vi "Main.vi"() -> ()   [LabVIEW 2013]
doc: "This template is for the Queued Message Handler design pattern.\n\nThe Event Handling Loop generates messages based on user interface actions.\n\nThe Message Handling Loop processes messages generated by the Event Handling Loop, or by other messages. The messages are string values, so new messages can be added easily to the Message Cases case structure in the Message Handling Loop. Each message cluster can also provide an optional value for Message Data, which is a variant that can be converted to whatever message-specific data is required."
uses:
  controls/UI Data.ctl
  <vilib>/vision/Image Controls.llb/IMAQ Image.ctl
  support/Message Queue/Message Queue.lvlib
  support/User Event - Stop/User Event - Stop.lvlib
  support/FPGA/FPGA Frame Grabbing.lvlib
  <vilib>/vision/NI_Vision_Development_Module.lvlib
  support/Image Processing/Image Processing.lvlib
panel:
  out "combo mask":T1(plugin-control)
  out "right \nannulus":T2 {"End Angle" format="%.2f"; "Start Angle" format="%.2f"; "Center X" scale=0.0..1024.0}
  out "right masked image":T1(plugin-control)
  out "right mask":T1(plugin-control)
  out "left annulus":T2 {"End Angle" format="%.2f"; "Start Angle" format="%.2f"; "Center X" scale=0.0..1024.0}
  out "left masked image":T1(plugin-control)
  out "left mask":T1(plugin-control)
  in  "Accept Threshold":bool
  in  "Threshold Range":cluster{"Lower value":dbl, "Upper value":dbl}={"Lower value"=0.0, "Upper value"=255.0} {"Upper value" min=0.0 max=255.0 scale=0.0..255.0; "Lower value" min=0.0 max=255.0 scale=0.0..255.0}
  out "FPGA image info":T5 {"Image Type" items=["Grayscale (U8)", "Grayscale (I16)", "Grayscale (SGL)", "Complex (CSG)", "RGB (U32)", "HSL (U32)", "RGB (U64)", "Grayscale (U16)"]}
  out "Processed Image":T1(plugin-control)
  in  "Stream?":bool
  out "FPGA Image":T1(plugin-control)
  in  "Save Mask Coordinates":bool
  in  "Test Visual Response":bool
  in  "Send Parameters to FPGA":bool
  out "Status Update":string="VI Stopped"
  in  "Define Mask":bool
  in  "Acquire Image":bool
  in  "Stop":bool
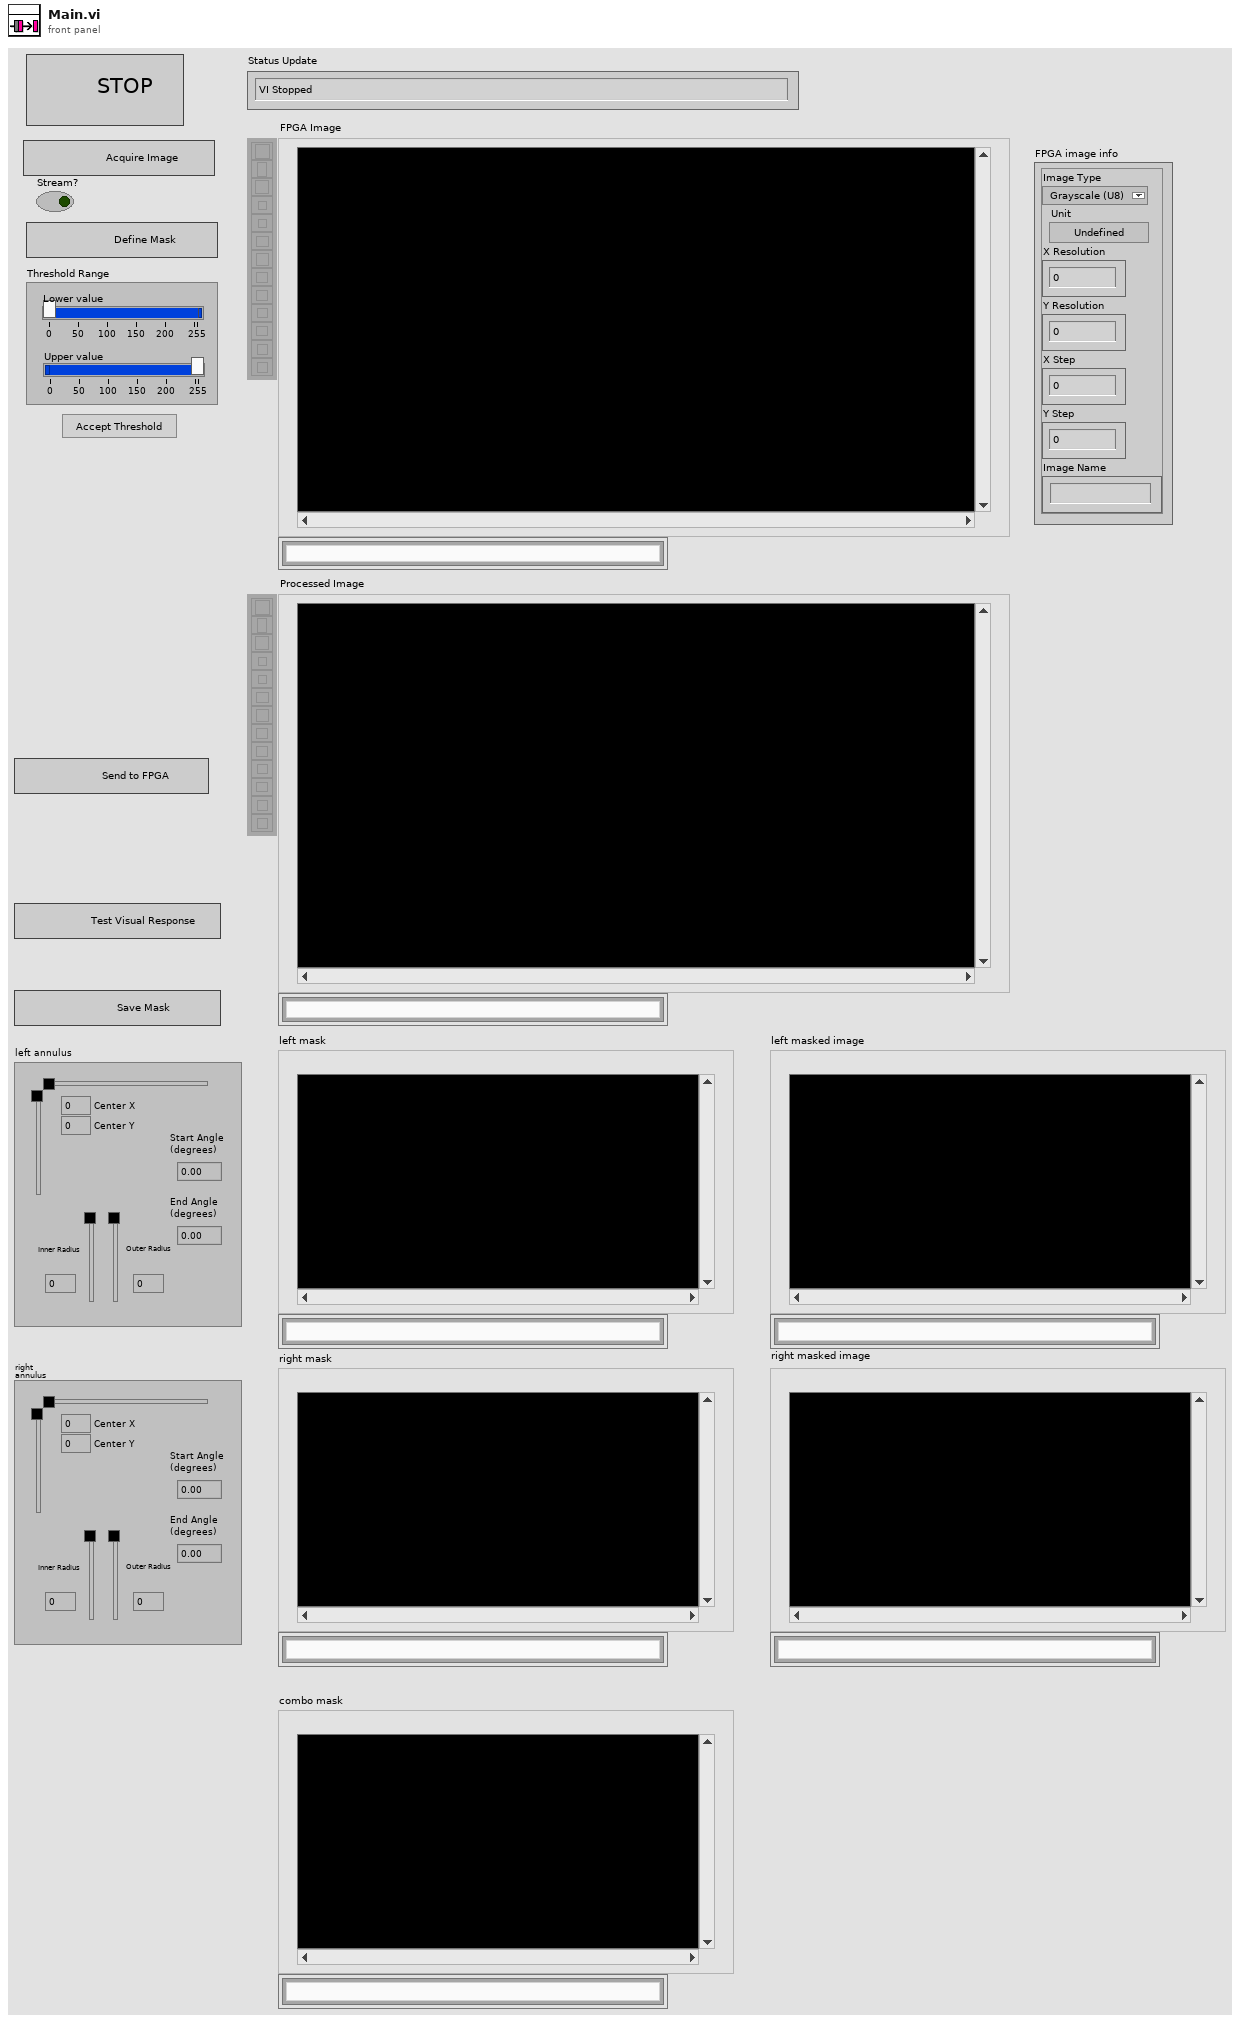
[diagram p1: front panel]
types:
  T1 = typedef "IMAQ Image.ctl" = refnum<image>
  T2 = typedef "IMAQ Circle" = cluster{"Center X":i32, "Center Y":i32, "Inner Radius":i32, "Outer Radius":i32, "Start Angle":dbl, "End Angle":dbl}
  T3 = typedef "Image Type" = u32
  T4 = typedef "Image Unit" = enum32{"Undefined", "Angström", "Micrometer", "Millimeter", "Centimeter", "Meter", "Kilometer", "Microinch", "Inch", "Feet", "Nautical miles", "Standard miles", "Steps"}
  T5 = cluster{"Image Type":T3, "Unit":T4, "X Resolution":i32, "Y Resolution":i32, "X Step":sgl, "Y Step":sgl, "Image Name":string}
  T6 = typedef "UI Data.ctl" = cluster{"Boolean <Replace Me>":bool, "Initial Message":string, "Numeric <Replace Me>":dbl, "Acquire Image Ref":refnum<vi>, "Define Mask Ref":refnum<vi>, "Status Update Ref":refnum<vi>, "Stop Button Ref":refnum<vi>, "FPGA Image":T1, "Processed Image":T1, "Left Annulus":cluster{"Center X":i32, "Center Y":i32, "Inner Radius":i32, "Outer Radius":i32, "Start Angle":dbl, "End Angle":dbl}, "Right Annulus":cluster{"Center X":i32, "Center Y":i32, "Inner Radius":i32, "Outer Radius":i32, "Start Angle":dbl, "End Angle":dbl}}
  T7 = typedef "Message Queue.lvlib/All Message Queues.ctl" = cluster{"UI":refnum<queue>}
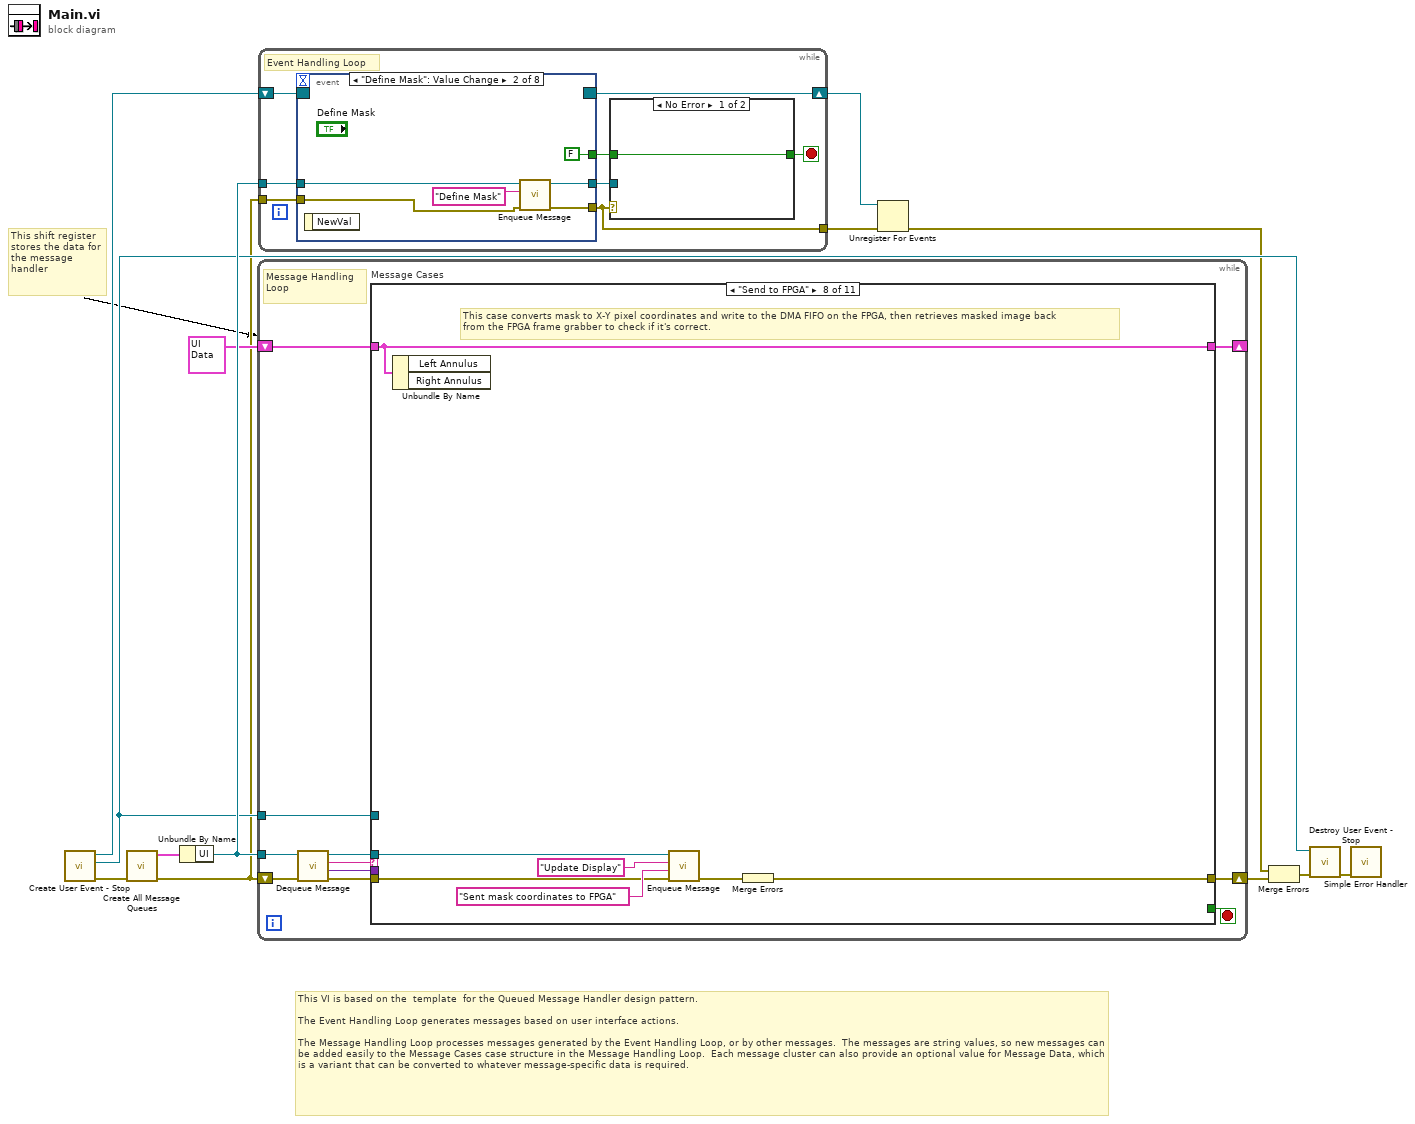
[diagram p0: block diagram]
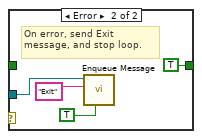
[diagram p2: hidden frame]
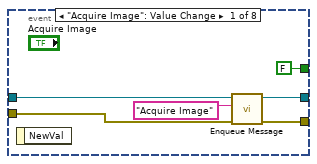
[diagram p3: hidden frame]
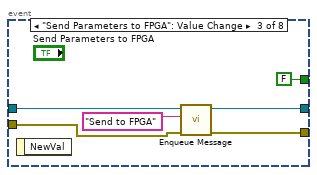
[diagram p4: hidden frame]
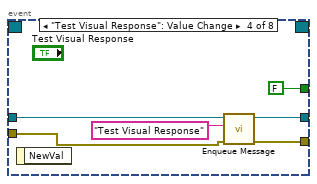
[diagram p5: hidden frame]
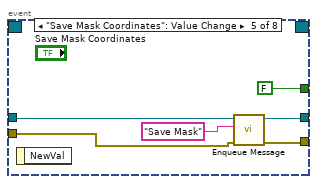
[diagram p6: hidden frame]
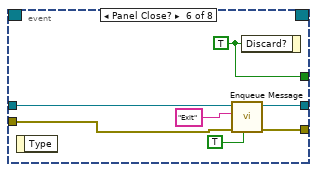
[diagram p7: hidden frame]
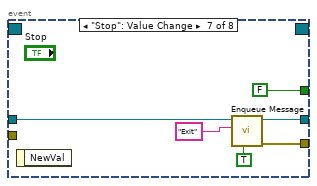
[diagram p8: hidden frame]
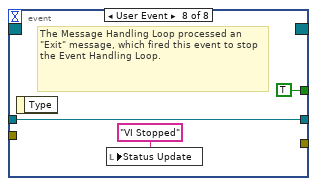
[diagram p9: hidden frame]
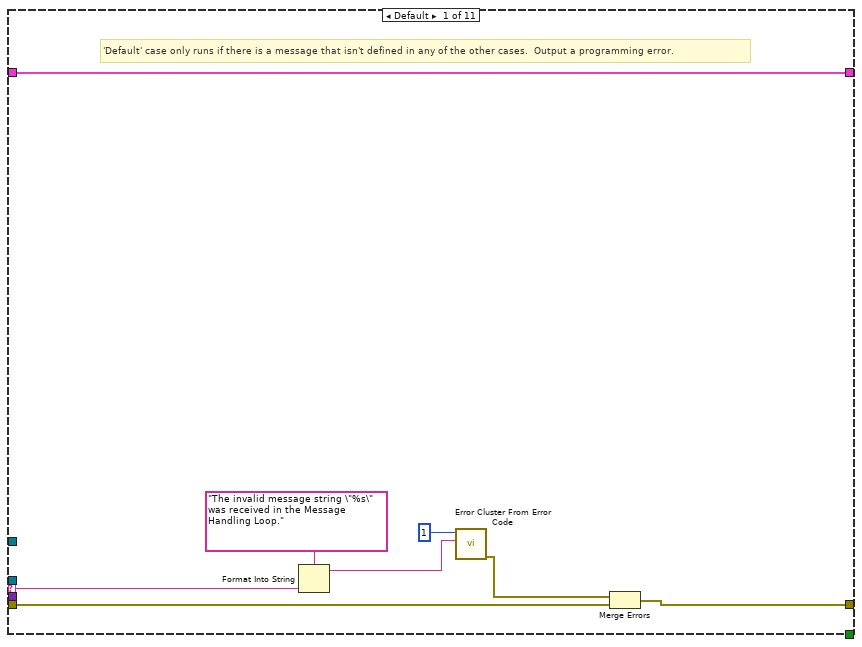
[diagram p10: hidden frame]
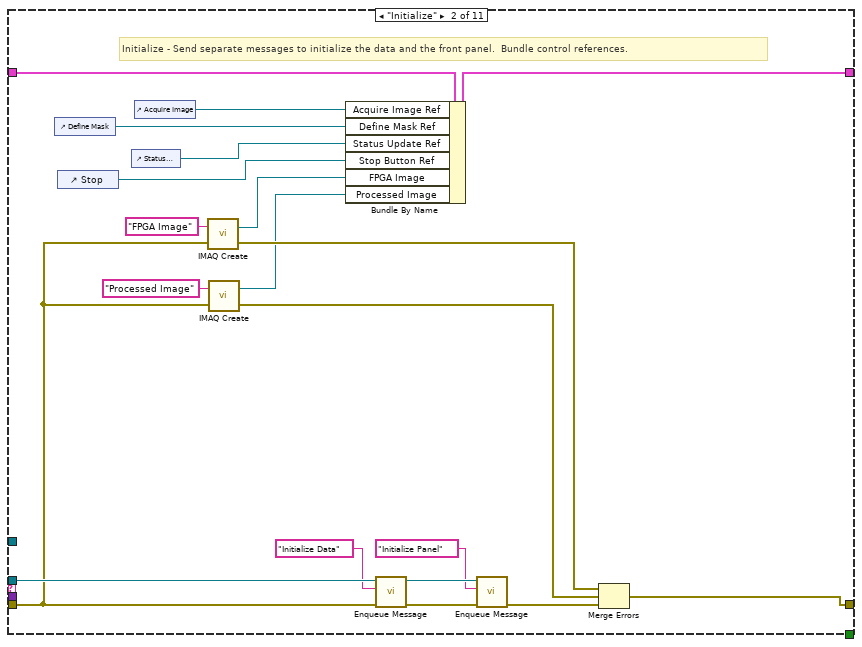
[diagram p11: hidden frame]
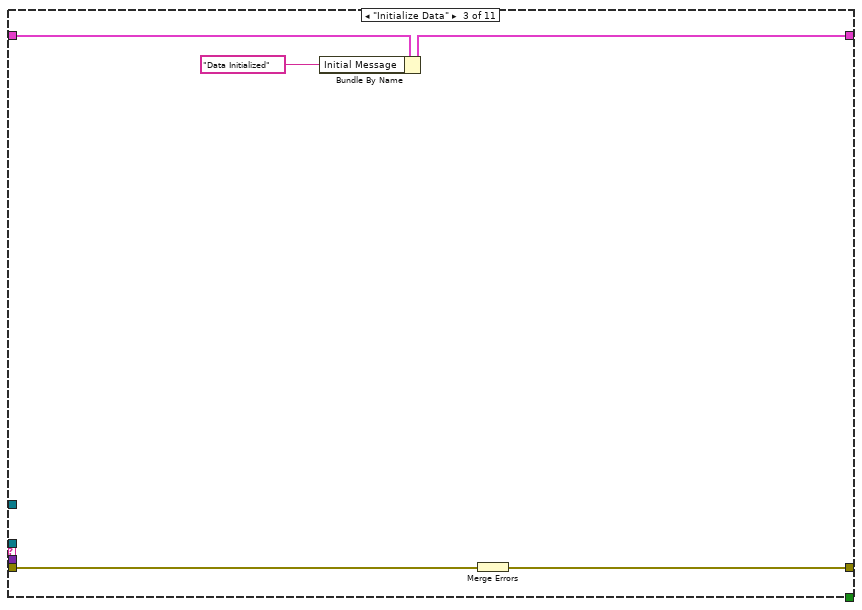
[diagram p12: hidden frame]
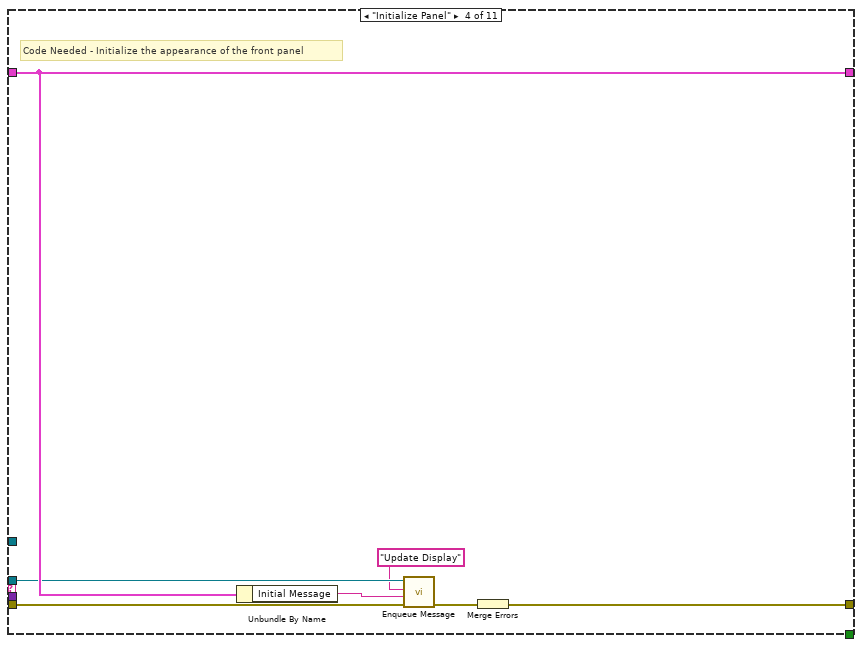
[diagram p13: hidden frame]
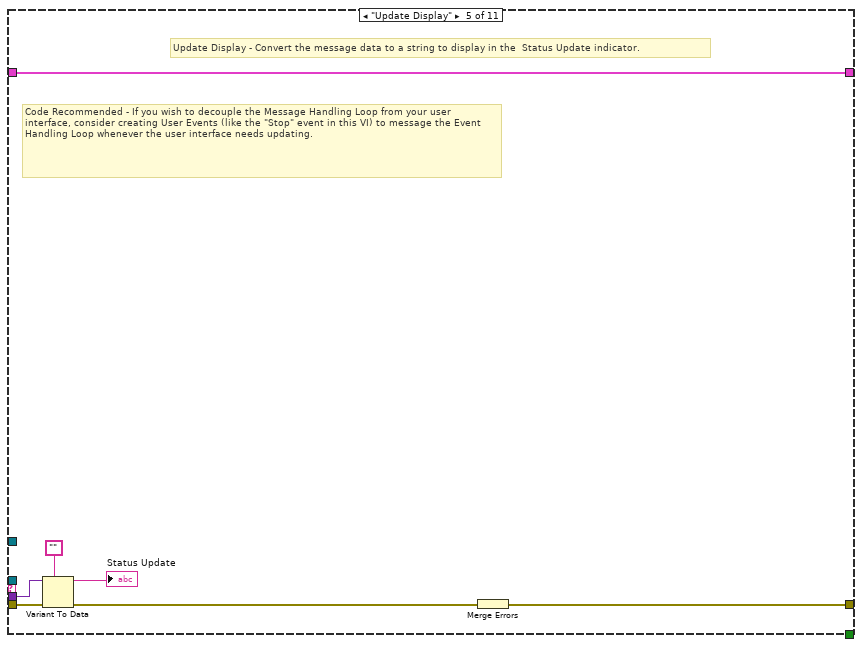
[diagram p14: hidden frame]
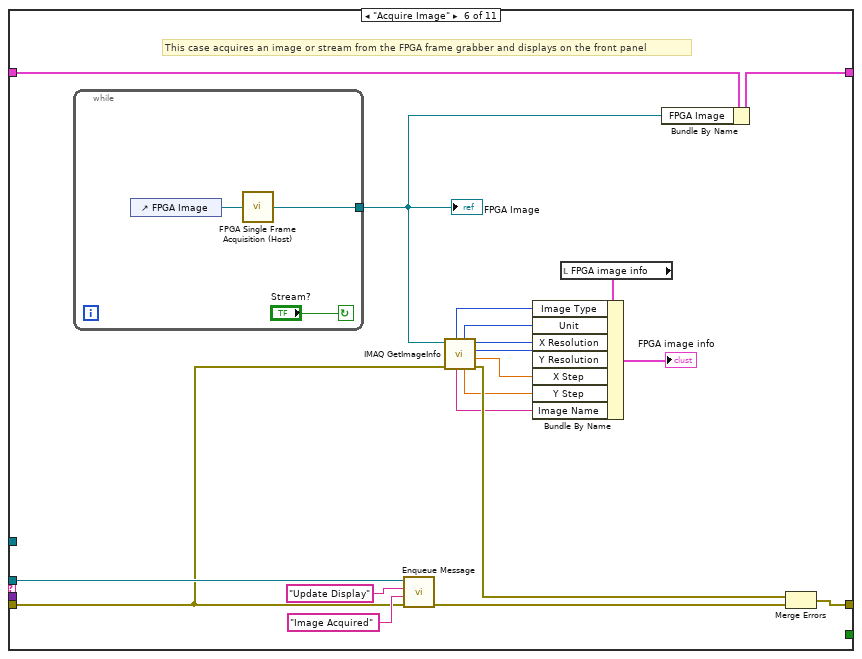
[diagram p15: hidden frame]
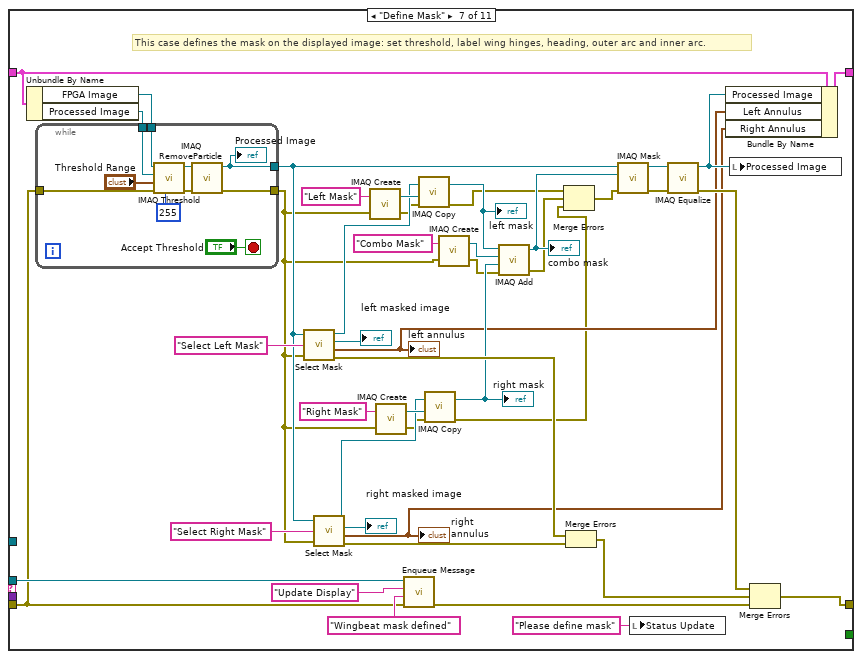
[diagram p16: hidden frame]
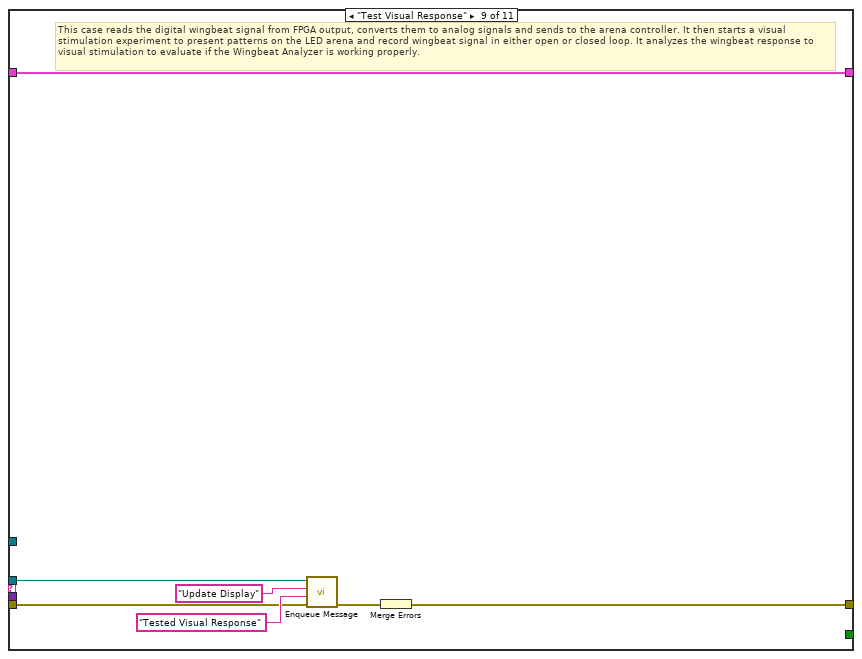
[diagram p17: hidden frame]
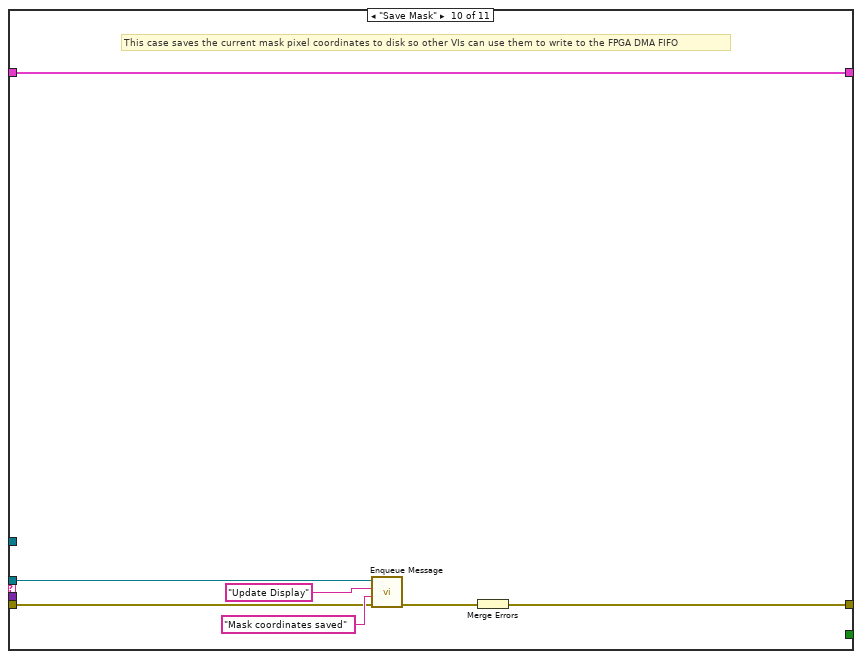
[diagram p18: hidden frame]
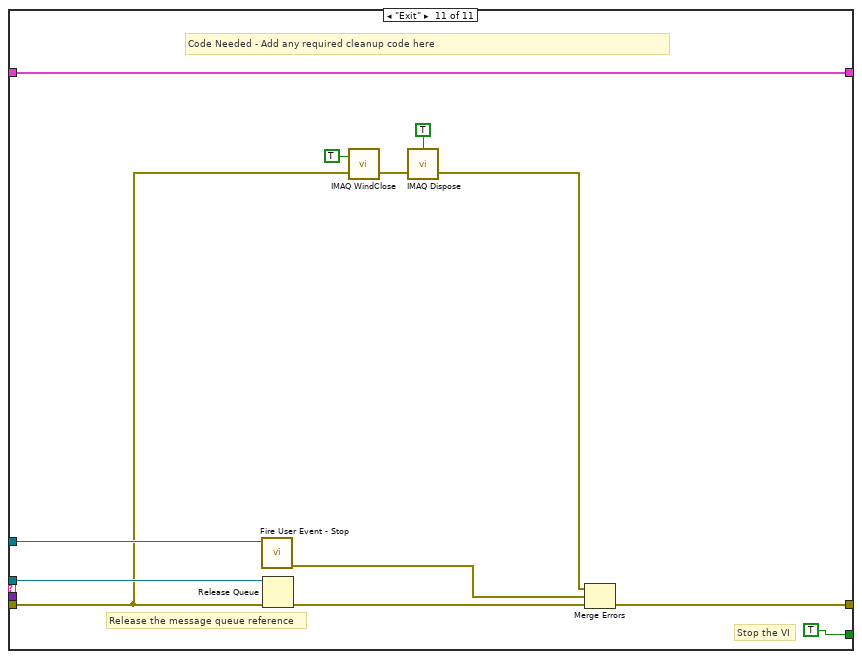
[diagram p19: hidden frame]
diagram:
  # "This VI is based on the  template  for the Queued Message Handler design pattern.\n\nThe Event Handling Loop generates messages based on user interface actions.\n\nThe Message Handling Loop processes messages generated by the Event Handling Loop, or by other messages.  The messages are string values, so new messages can be added easily to the Message Cases case structure in the Message Handling Loop.  Each message cluster can also provide an optional value for Message Data, which is a variant that can be converted to whatever message-specific data is required."
  # "This shift register\nstores the data for the message handler"
  n1 = call "Create User Event - Stop.vi"() -> ("error out"=w9:errorcluster, "User Event - Stop"=w6:refnum<user-event>, "Stop Event Registration Refnum"=w10:refnum<event-registration>)  [unwired: 9 in]
  n2 = call "Create All Message Queues.vi"("error in (no error)"=w9) -> ("error out"=w1:errorcluster, "Message Queues out"=w13:T7)  [unwired: 9 in]
  n3 = Unbundle By Name(w13) -> ("UI"=w11:refnum<queue>)
  n4 = while {
    tunnel: w11 -> [w14]
    shift-right: [w23] -> _
    shift-left: T6 {"Boolean <Replace Me>"=TRUE, "Initial Message"="", "Numeric <Replace Me>"=0.0, "Acquire Image Ref"=refnum, "Define Mask Ref"=refnum, "Status Update Ref"=refnum, "Stop Button Ref"=refnum, "FPGA Image"=refnum, "Processed Image"=refnum, "Left Annulus"={"Center X"=0, "Center Y"=0, "Inner Radius"=0, "Outer Radius"=0, "Start Angle"=0.0, "End Angle"=0.0}, "Right Annulus"={"Center X"=0, "Center Y"=0, "Inner Radius"=0, "Outer Radius"=0, "Start Angle"=0.0, "End Angle"=0.0}} ("Data Cluster") -> [w24]
    tunnel: w6 -> [w20]
    shift-right: [w21] -> w12
    shift-left: w1 -> [w19]
    stop <- w22 stop-if-true
    # "Message Handling Loop"
    n5 = call "Dequeue Message.vi"("error in (no error)"=w19, "Message Queue"=w14) -> ("error out"=w18:errorcluster, "Message Data"=w16:variant, "Message"=w17:string, "dup Message Queue"=w15:refnum<queue>)  [unwired: 6 in]
    n6 = case "Message Cases" shown="\"Send to FPGA\"" w17 {
      selector: w17 -> [w30 _ _ _ _ _ _ _ _ _ _]
      tunnel: w15 -> [_ w50 _ w61 _ w88 w137 w150 w156 w164 w180]
      tunnel: w18 -> [w27 w35 w57 w62 w69 w83 w134 w151 w157 w162 w169]
      tunnel: [w25 w37 w53 w63 w70 w90 w94 w149 w155 w167 w176] -> w21
      tunnel: w24 -> [w32 w47 w56 w64 w71 w85 w133 w148 w161 w168 w179]
      tunnel: [w32 w46 w55 w64 w71 w84 w132 w148 w161 w168 w179] -> w23
      tunnel: [_ _ _ _ _ _ _ _ _ _ TRUE] -> w22
      tunnel: w16 -> [_ _ _ _ w68 _ _ _ _ _ _]
      tunnel: w20 -> [_ _ _ _ _ _ _ _ _ _ w175]
      frame Default {
        # "'Default' case only runs if there is a message that isn't defined in any of the other cases.  Output a programming error."
        n7 = Format Into String(format string="The invalid message string \"%s\" was received in the Message Handling Loop." ("Unknown Message Error Text"), w30) -> (resulting string=w28:string)  [unwired: 2 in, 1 out]
        n8 = call <vilib>:"Error Cluster From Error Code.vi"("error message (\"\")"=w28, "error code (0)"=1) -> ("error out"=w26:errorcluster)  [unwired: 7 in]
        n9 = Merge Errors(w26, w27) -> (w25:errorcluster)
      }
      frame "Initialize" {
        # "Initialize - Send separate messages to initialize the data and the front panel.  Bundle control references."
        n10 = control-ref of="Define Mask"() -> (w44:refnum<vi>)
        n11 = control-ref of="Stop"() -> (w42:refnum<vi>)
        n12 = control-ref of="Status Update"() -> (w43:refnum<vi>)
        n13 = control-ref of="Acquire Image"() -> (w45:refnum<vi>)
        n14 = call "IMAQ Create"("Image Name"="FPGA Image", "error in (no error)"=w35) -> ("New Image"=w40:T1, "error out"=w36:errorcluster)  [unwired: 3 in]
        n15 = call "IMAQ Create"("Image Name"="Processed Image", "error in (no error)"=w35) -> ("New Image"=w33:T1, "error out"=w34:errorcluster)  [unwired: 3 in]
        n16 = Bundle By Name(cluster=w47, "Acquire Image Ref"=w45, "Define Mask Ref"=w44, "Status Update Ref"=w43, "Stop Button Ref"=w42, "FPGA Image"=w40, "Processed Image"=w33) -> (w46:T6)
        n17 = call "Enqueue Message.vi"("error in (no error)"=w35, "Message"="Initialize Data", "Message Queue"=w50) -> ("error out"=w52:errorcluster, "dup Message Queue"=w51:refnum<queue>)  [unwired: 7 in]
        n18 = call "Enqueue Message.vi"("error in (no error)"=w52, "Message"="Initialize Panel", "Message Queue"=w51) -> ("error out"=w38:errorcluster)  [unwired: 7 in, 1 out]
        n19 = Merge Errors(w36, w34, w38) -> (w37:errorcluster)
      }
      frame "Initialize Data" {
        n20 = Bundle By Name(cluster=w56, "Initial Message"="Data Initialized") -> (w55:T6)
        n21 = Merge Errors(w57) -> (w53:errorcluster)
      }
      frame "Initialize Panel" {
        # "Code Needed - Initialize the appearance of the front panel"
        n22 = Unbundle By Name(w64) -> ("Initial Message"=w58:string)
        n23 = call "Enqueue Message.vi"("error in (no error)"=w62, "Message Data"=w58, "Message"="Update Display", "Message Queue"=w61) -> ("error out"=w60:errorcluster)  [unwired: 6 in, 1 out]
        n24 = Merge Errors(w60) -> (w63:errorcluster)
      }
      frame "Update Display" {
        # "Code Recommended - If you wish to decouple the Message Handling Loop from your user interface, consider creating User Events (like the \"Stop\" event in this VI) to message the Event Handling Loop whenever the user interface needs updating."
        # "Update Display - Convert the message data to a string to display in the  Status Update indicator."
        n25 = Variant To Data(error in=w69, type="", Variant=w68) -> (data=→"Status Update":string, error out=w66:errorcluster)
        n26 = Merge Errors(w66) -> (w70:errorcluster)
      }
      frame "Acquire Image" {
        # "This case acquires an image or stream from the FPGA frame grabber and displays on the front panel"
        n27 = while {
          tunnel: [w92] -> w72
          stop <- "Stream?" continue-if-true
          n28 = control-ref of="FPGA Image"() -> (w91:refnum<vi>)
          n29 = call "FPGA Single Frame Acquisition (Host).vi"("Ctl Refnum"=w91) -> ("Image"=w92:T1)
        }
        "FPGA Image" <- w72
        n30 = call "Enqueue Message.vi"("error in (no error)"=w83, "Message Data"="Image Acquired" ("\"Do Something\" button pressed"), "Message"="Update Display", "Message Queue"=w88) -> ("error out"=w89:errorcluster)  [unwired: 6 in, 1 out]
        n31 = call "IMAQ GetImageInfo"("error in (no error)"=w83, "Image"=w72) -> ("error out"=w82:errorcluster, "X Step"=w77:sgl, "Y Resolution"=w78:i32, "X Resolution"=w79:i32, "Y Step"=w76:sgl, "Unit"=w80:T4, "Image Name"=w75:string, "Image Type"=w81:T3)  [unwired: 2 in]
        n32 = local read "FPGA image info"() -> (w73:T5)
        n33 = Bundle By Name(cluster=w73, "Image Type"=w81, "Unit"=w80, "X Resolution"=w79, "Y Resolution"=w78, "X Step"=w77, "Y Step"=w76, "Image Name"=w75) -> (→"FPGA image info":T5)
        n34 = Bundle By Name(cluster=w85, "FPGA Image"=w72) -> (w84:T6)
        n35 = Merge Errors(w82, w89) -> (w90:errorcluster)
      }
      frame "Define Mask" {
        # "This case defines the mask on the displayed image: set threshold, label wing hinges, heading, outer arc and inner arc."
        n36 = Unbundle By Name(w133) -> ("FPGA Image"=w131:T1, "Processed Image"=w130:T1)
        n37 = while {
          tunnel: w134 -> [w147]
          tunnel: w131 -> [w146]
          tunnel: w130 -> [w145]
          tunnel: [w138] -> w116
          tunnel: [w140] -> w100
          stop <- "Accept Threshold" stop-if-true
          n38 = call "IMAQ Threshold"("Replace Value"=u8 255, "error in (no error)"=w147, "Range"="Threshold Range", "Image Dst"=w145, "Image Src"=w146) -> ("error out"=w143:errorcluster, "Image Dst Out"=w142:T1)  [unwired: 1 in, 4 out]
          n39 = call "IMAQ RemoveParticle"("error in (no error)"=w143, "Image Src"=w142) -> ("error out"=w140:errorcluster, "Image Dst Out"=w138:T1)  [unwired: 5 in, 3 out]
          "Processed Image" <- w138
        }
        n40 = call "Select Mask.vi"("Read \nImage"=w116, "Prompt"="Select Left Mask", "error in"=w100) -> ("mask"=w109:T1, "Masked \nImage"=→"left masked image":T1, "Annulus"=w105:T2, "error out"=w120:errorcluster)  [unwired: 1 out]
        "left annulus" <- w105
        n41 = call "Select Mask.vi"("Read \nImage"=w116, "Prompt"="Select Right Mask", "error in"=w100) -> ("mask"=w107:T1, "Masked \nImage"=→"right masked image":T1, "Annulus"=w104:T2, "error out"=w119:errorcluster)  [unwired: 1 out]
        "right \nannulus" <- w104
        n42 = call "IMAQ Create"("Image Name"="Left Mask", "error in (no error)"=w100) -> ("New Image"=w112:T1, "error out"=w103:errorcluster)  [unwired: 3 in]
        n43 = call "IMAQ Create"("Image Name"="Right Mask", "error in (no error)"=w100) -> ("New Image"=w110:T1, "error out"=w102:errorcluster)  [unwired: 3 in]
        n44 = call "Enqueue Message.vi"("error in (no error)"=w134, "Message Data"="Wingbeat mask defined" ("\"Do Something Else\" button pressed"), "Message"="Update Display", "Message Queue"=w137) -> ("error out"=w95:errorcluster)  [unwired: 6 in, 1 out]
        n45 = call "IMAQ Copy"("error in (no error)"=w103, "Image Dst"=w112, "Image Src"=w109) -> ("error out"=w99:errorcluster, "Image Dst Out"=w108:T1)  [unwired: 3 in]
        "left mask" <- w108
        n46 = call "IMAQ Copy"("error in (no error)"=w102, "Image Dst"=w110, "Image Src"=w107) -> ("error out"=w97:errorcluster, "Image Dst Out"=w106:T1)  [unwired: 3 in]
        "right mask" <- w106
        n47 = call "IMAQ Create"("Image Name"="Combo Mask", "error in (no error)"=w100) -> ("New Image"=w117:T1, "error out"=w101:errorcluster)  [unwired: 3 in]
        n48 = call "IMAQ Add"("Image Src A"=w108, "Image Dst"=w117, "Image Src B"=w106, "error in (no error)"=w101) -> ("Image Dst Out"=w114:T1, "error out"=w98:errorcluster)  [unwired: 3 in]
        "combo mask" <- w114
        n49 = Merge Errors(w99, w98, w97) -> (w96:errorcluster)
        n50 = Merge Errors(w120, w119) -> (w115:errorcluster)
        n51 = call "IMAQ Mask"("error in (no error)"=w96, "Image Mask"=w114, "Image Src"=w116) -> ("error out"=w125:errorcluster, "Image Dst Out"=w126:T1)  [unwired: 1 in, 1 out]
        n52 = local write "Status Update"("Please define mask" ("Status Update")) -> ()
        n53 = call "IMAQ Equalize"("error in (no error)"=w125, "Image Src"=w126) -> ("error out"=w128:errorcluster, "Image Dst Out"=w124:T1)  [unwired: 4 in, 4 out]
        n54 = Bundle By Name(cluster=w133, "Processed Image"=w124, "Left Annulus"=w105, "Right Annulus"=w104) -> (w132:T6)
        n55 = local write "Processed Image"(w124) -> ()
        n56 = Merge Errors(w128, w115, w95) -> (w94:errorcluster)
      }
      frame "Send to FPGA" {
        # "This case converts mask to X-Y pixel coordinates and write to the DMA FIFO on the FPGA, then retrieves masked image back \nfrom the FPGA frame grabber to check if it's correct."
        n57 = Unbundle By Name(w148) -> ()  [unwired: 2 out]
        n58 = call "Enqueue Message.vi"("error in (no error)"=w151, "Message Data"="Sent mask coordinates to FPGA" ("\"Do Something\" button pressed"), "Message"="Update Display", "Message Queue"=w150) -> ("error out"=w154:errorcluster)  [unwired: 6 in, 1 out]
        n59 = Merge Errors(w154) -> (w149:errorcluster)
      }
      frame "Test Visual Response" {
        # "This case reads the digital wingbeat signal from FPGA output, converts them to analog signals and sends to the arena controller. It then starts a visual stimulation experiment to present patterns on the LED arena and record wingbeat signal in either open or closed loop. It analyzes the wingbeat response to visual stimulation to evaluate if the Wingbeat Analyzer is working properly."
        n60 = call "Enqueue Message.vi"("error in (no error)"=w157, "Message Data"="Tested Visual Response" ("\"Do Something\" button pressed"), "Message"="Update Display", "Message Queue"=w156) -> ("error out"=w160:errorcluster)  [unwired: 6 in, 1 out]
        n61 = Merge Errors(w160) -> (w155:errorcluster)
      }
      frame "Save Mask" {
        # "This case saves the current mask pixel coordinates to disk so other VIs can use them to write to the FPGA DMA FIFO"
        n62 = call "Enqueue Message.vi"("error in (no error)"=w162, "Message Data"="Mask coordinates saved" ("\"Do Something Else\" button pressed"), "Message"="Update Display", "Message Queue"=w164) -> ("error out"=w163:errorcluster)  [unwired: 6 in, 1 out]
        n63 = Merge Errors(w163) -> (w167:errorcluster)
      }
      frame "Exit" {
        # "Stop the VI"
        # "Release the message queue reference"
        # "Code Needed - Add any required cleanup code here"
        n64 = call "Fire User Event - Stop.vi"("User Event - Stop"=w175) -> ("error out"=w174:errorcluster)  [unwired: 10 in]
        n65 = Release Queue(queue=w180, error in (no error)=w169) -> (error out=w177:errorcluster)  [unwired: 1 in, 2 out]
        n66 = call "IMAQ WindClose"("Close All Windows (False)"=TRUE, "error in (no error)"=w169) -> ("error out"=w171:errorcluster)  [unwired: 4 in]
        n67 = call "IMAQ Dispose"("All Images? (No)"=TRUE, "error in (no error)"=w171) -> ("error out"=w170:errorcluster)  [unwired: 4 in]
        n68 = Merge Errors(w170, w174, w177) -> (w176:errorcluster)
      }
    }
  }
  n69 = while {
    tunnel: w11 -> [w188]
    tunnel: [w184] -> w4
    shift-right: [w182] -> w3
    shift-left: w10 -> [w183]
    tunnel: w1 -> [w181]
    stop <- w186 stop-if-true
    # "Event Handling Loop"
    n70 = event shown="[1] \"Define Mask\": Value Change" {
      selector: w183 -> [_ _ _ _ _ _ _ _]
      dyn-events: [_ _ _ _ _ _ _ _] -> w182
      timeout: _ -> [_ _ _ _ _ _ _ _]
      tunnel: [FALSE ("Discard?") FALSE ("Discard?") FALSE ("Discard?") FALSE ("Discard?") FALSE ("Discard?") w230 FALSE ("Discard?") TRUE ("Discard?")] -> w187
      tunnel: w188 -> [w199 w205 w211 w216 w221 w229 w236 w239]
      tunnel: [w198 w203 w208 w213 w218 w228 w235 _] -> w184
      tunnel: [w197 w204 w207 w215 w220 w227 w233 w239] -> w185
      tunnel: w181 -> [w195 w201 w209 w212 w219 w224 _ _]
      event "Acquire Image": Value Change {
        n71 = event-data() -> ()  [unwired: 1 in, 1 out]
        n72 = call "Enqueue Message.vi"("error in (no error)"=w195, "Message"="Acquire Image", "Message Queue"=w199) -> ("error out"=w198:errorcluster, "dup Message Queue"=w197:refnum<queue>)  [unwired: 7 in]
      }
      event "Define Mask": Value Change {
        n73 = event-data() -> ()  [unwired: 1 in, 1 out]
        n74 = call "Enqueue Message.vi"("error in (no error)"=w201, "Message"="Define Mask", "Message Queue"=w205) -> ("error out"=w203:errorcluster, "dup Message Queue"=w204:refnum<queue>)  [unwired: 7 in]
      }
      event "Send Parameters to FPGA": Value Change {
        n75 = event-data() -> ()  [unwired: 1 in, 1 out]
        n76 = call "Enqueue Message.vi"("error in (no error)"=w209, "Message"="Send to FPGA", "Message Queue"=w211) -> ("error out"=w208:errorcluster, "dup Message Queue"=w207:refnum<queue>)  [unwired: 7 in]
      }
      event "Test Visual Response": Value Change {
        n77 = event-data() -> ()  [unwired: 1 in, 1 out]
        n78 = call "Enqueue Message.vi"("error in (no error)"=w212, "Message"="Test Visual Response", "Message Queue"=w216) -> ("error out"=w213:errorcluster, "dup Message Queue"=w215:refnum<queue>)  [unwired: 7 in]
      }
      event "Save Mask Coordinates": Value Change {
        n79 = event-data() -> ()  [unwired: 1 in, 1 out]
        n80 = call "Enqueue Message.vi"("error in (no error)"=w219, "Message"="Save Mask", "Message Queue"=w221) -> ("error out"=w218:errorcluster, "dup Message Queue"=w220:refnum<queue>)  [unwired: 7 in]
      }
      event Panel Close? {
        w230 = TRUE ("Discard?")
        n81 = event-data() -> ()  [unwired: 1 in, 1 out]
        n82 = call "Enqueue Message.vi"("Priority Message? (F)"=TRUE, "error in (no error)"=w224, "Message"="Exit", "Message Queue"=w229) -> ("error out"=w228:errorcluster, "dup Message Queue"=w227:refnum<queue>)  [unwired: 6 in]
        n83 = event-data("Discard?"=w230) -> ()  [unwired: 1 in, 1 out]
      }
      event "Stop": Value Change {
        n84 = event-data() -> ()  [unwired: 1 in, 1 out]
        n85 = call "Enqueue Message.vi"("Priority Message? (F)"=TRUE, "Message"="Exit", "Message Queue"=w236) -> ("error out"=w235:errorcluster, "dup Message Queue"=w233:refnum<queue>)  [unwired: 7 in]
      }
      event User Event {
        # "The Message Handling Loop processed an \"Exit\" message, which fired this event to stop the Event Handling Loop."
        n86 = event-data() -> ()  [unwired: 1 in, 1 out]
        n87 = local write "Status Update"("VI Stopped" ("VI Stopped")) -> ()
      }
    }
    n88 = case shown="No Error" w184 {
      tunnel: [w189 TRUE ("Discard?")] -> w186
      tunnel: w187 -> [w189 _]
      tunnel: w185 -> [_ w192]
      frame No Error {
      }
      frame Error {
        # "On error, send Exit message, and stop loop."
        n89 = call "Enqueue Message.vi"("Priority Message? (F)"=TRUE, "Message"="Exit", "Message Queue"=w192) -> ()  [unwired: 7 in, 2 out]
      }
    }
  }
  n90 = Unregister For Events(event registration refnum=w3, error in=w4) -> (error out=w5:errorcluster)
  n91 = Merge Errors(w5, w12) -> (w7:errorcluster)
  n92 = call "Destroy User Event - Stop.vi"("error in (no error)"=w7, "User Event - Stop"=w6) -> ("error out"=w8:errorcluster)  [unwired: 9 in]
  n93 = call <vilib>:"Simple Error Handler.vi"("error in (no error)"=w8) -> ()  [unwired: 4 in, 5 out]
